vi "Create Tiger.vi"() -> (3 "output cluster":refnum<class "Tiger.lvclass">)   [LabVIEW 2018, in "Tiger.lvclass"]
uses:
  Tiger.lvclass
  Tiger.lvclass/Tiger.ctl
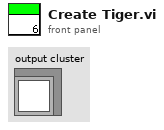
[diagram p1: front panel]
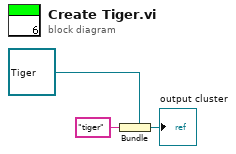
[diagram p0: block diagram]
diagram:
  n1 = Bundle(cluster=refnum<class "Tiger.lvclass"> refnum ("Tiger.lvclass"), "tiger" ("String")) -> (→"output cluster":refnum<class "Tiger.lvclass">)
